vi "SWERVE DRIVE AUTO.vi"(8 "error in (no error)":errorcluster, 11 "auto pgm array":T4[](array[typedef])=[{"auto drive command"={"TRANSLATE"={"drive\ndistance (ft)"=10.0, "steer\nbearing (deg)"=0.0, "max strafe\nvelocity (ft/s)"=10.0, "max strafe\naccel (ft/s^2)"=58.7}, "ROTATE"={"rotate to\nbearing (deg)"=0.0, "max rotate\nvelocity (deg/s)"=0.0, "max rotate\naccel (ft/s^2)"=25.0}}, "sub-systems"={"start INTAKE"=FALSE, "extend FLAP"=FALSE, "SHOOT"=FALSE, "retract FLAP"=FALSE, "TARGET SPEAKER"=FALSE, "TARGET AMP"=FALSE, "TARGET OFF"=FALSE, "DANCE"=FALSE}}, {"auto drive command"={"TRANSLATE"={"drive\ndistance (ft)"=5.0, "steer\nbearing (deg)"=180.0, "max strafe\nvelocity (ft/s)"=5.0, "max strafe\naccel (ft/s^2)"=58.7}, "ROTATE"={"rotate to\nbearing (deg)"=0.0, "max rotate\nvelocity (deg/s)"=180.0, "max rotate\naccel (ft/s^2)"=25.0}}, "sub-systems"={"start INTAKE"=FALSE, "extend FLAP"=FALSE, "SHOOT"=FALSE, "retract FLAP"=FALSE, "TARGET SPEAKER"=FALSE, "TARGET AMP"=FALSE, "TARGET OFF"=FALSE, "DANCE"=FALSE}}] {"auto drive command"."ROTATE"."max rotate\naccel (ft/s^2)" min=0.0 max=200.0 step=0.1 format="%_3f"; "auto drive command"."ROTATE"."max rotate\nvelocity (deg/s)" min=0.0 step=0.001; "auto drive command"."TRANSLATE"."max strafe\naccel (ft/s^2)" min=0.0 max=200.0 step=0.1 format="%_3f"; "auto drive command"."TRANSLATE"."max strafe\nvelocity (ft/s)" min=0.0 max=20.0 step=0.001 format="%_5f"}) -> (0 "error out":errorcluster)   [LabVIEW 2023]
uses:
  ctrl defs/ctrl AUTONOMOUS step control.ctl
  ctrl defs/ctrl AUTONOMOUS drive step control.ctl
  ctrl defs/ctrl AUTONOMOUS systems step control.ctl
  ctrl defs/ctrl AUTO STATES.ctl
  <vilib>/Rock Robotics/WPI/ThirdParty/REV Robotics/REVLib/Typedef/Spark MAX Smart Motion Parameters.ctl
  <vilib>/Rock Robotics/WPI/ThirdParty/REV Robotics/REVLib/Typedef/Spark MAX Control Type.ctl
  Global INIT.vi
  Global odometry.vi
  <vilib>/Rock Robotics/WPI/ThirdParty/Phoenix-LabVIEW/CANCoder/Get/CTRE_Phoenix_CANcoder_GetSensorData.vi
  Global stack names.vi
  <vilib>/Rock Robotics/Network Tables/NT Read Boolean.vi
  <vilib>/Rock Robotics/Network Tables/NT Write Boolean.vi
panel:
  out "Sensor Velocity":dbl[](array[numeric])
  in  "Smart Motion Parameters":T1
  in  "PID Constants":T2={"P Gain"=0.0, "I Gain"=0.0, "D Gain"=0.0, "F Gain"=0.0, "I Zone"=0.0, "Min Output"=-1.0, "Max Output"=1.0} {"Max Output" min=0.0 max=1.0 step=0.01; "Min Output" min=-1.0 max=0.0 step=0.01}
  in  "loop exit":bool
  in  "STATE":T3
  out "wheel\npos (rev)":dbl[](array[numeric])
  out "@ target":bool[](array[boolean])
  out "pos\ntarget (rev)":dbl[](array[numeric])
  out "rev tol\nto target":dbl
  out "distance (ft)\nto wheel revs":dbl
  out "vel to wheel\nspeed\n(rpm per ft/s)":dbl
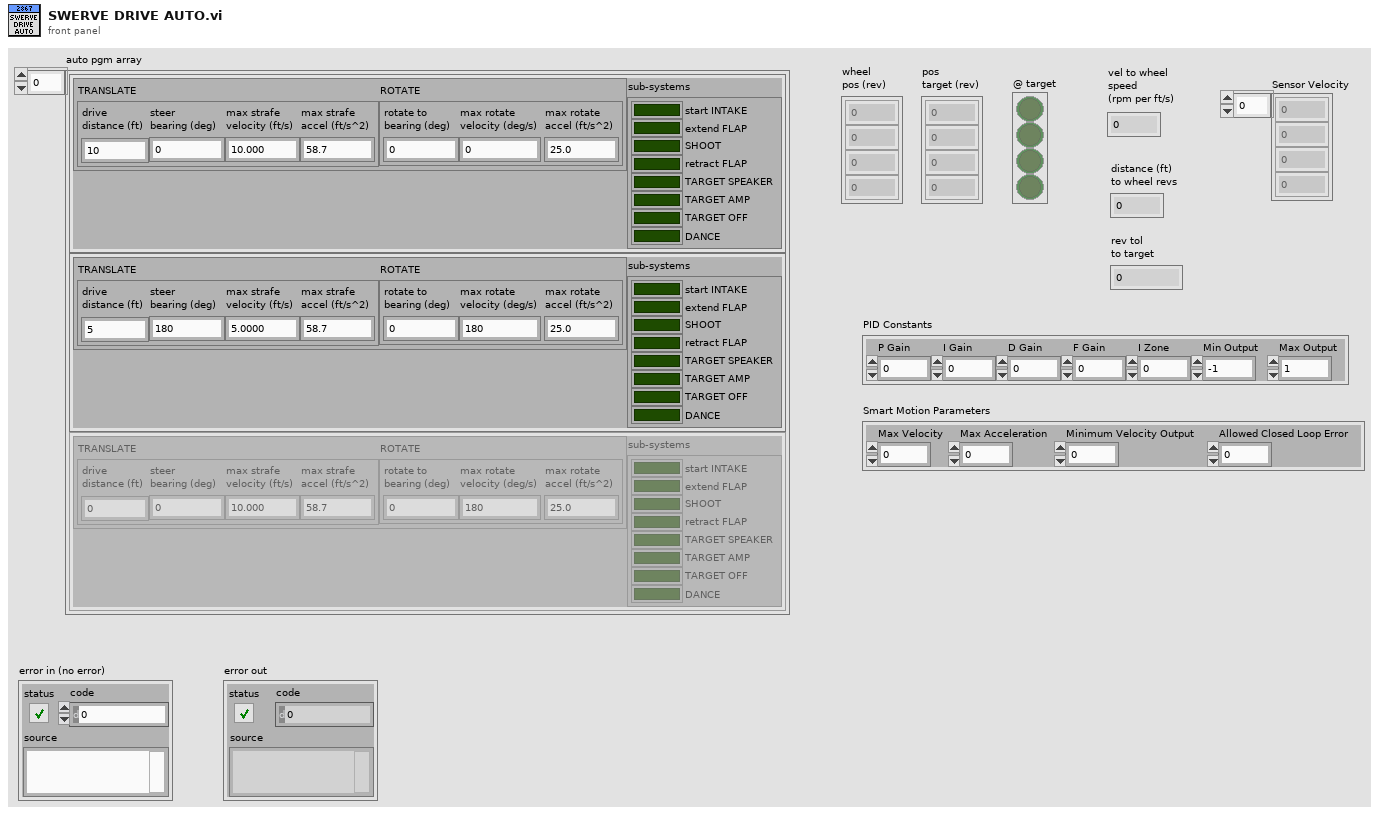
[diagram p1: front panel]
types:
  T1 = typedef "Spark MAX Smart Motion Parameters.ctl" = cluster{"Max Velocity":dbl, "Max Acceleration":dbl, "Minimum Velocity Output":dbl, "Allowed Closed Loop Error":dbl}
  T2 = cluster{"P Gain":dbl, "I Gain":dbl, "D Gain":dbl, "F Gain":dbl, "I Zone":dbl, "Min Output":dbl, "Max Output":dbl}
  T3 = typedef "ctrl AUTO STATES.ctl" = enum16{"TRANSLATE", "ROTATE", "TARGET", "INTAKE", "SHOOT", "DANCE", "WAIT for INTAKE", "WAIT for SHOOTER", "END", "SUB-SYSTEMS"}
  T4 = typedef "ctrl AUTONOMOUS step control.ctl" = cluster{"auto drive command":T5, "sub-systems":T6}
  T5 = typedef "ctrl AUTONOMOUS drive step control.ctl" = cluster{"TRANSLATE":cluster{"drive\ndistance (ft)":dbl, "steer\nbearing (deg)":dbl, "max strafe\nvelocity (ft/s)":dbl, "max strafe\naccel (ft/s^2)":dbl}, "ROTATE":cluster{"rotate to\nbearing (deg)":dbl, "max rotate\nvelocity (deg/s)":dbl, "max rotate\naccel (ft/s^2)":dbl}}
  T6 = typedef "ctrl AUTONOMOUS systems step control.ctl" = cluster{"start INTAKE":bool, "extend FLAP":bool, "SHOOT":bool, "retract FLAP":bool, "TARGET SPEAKER":bool, "TARGET AMP":bool, "TARGET OFF":bool, "DANCE":bool}
  T7 = typedef "ctrl swerve motor.ctl" = cluster{"description":string, "MOTOR SELECT":T8, "Installed?":bool, "CAN ID":u8, "refnum name":string, "Invert":bool, "Idle Mode":T9, "Current limiting":T10, "MOTOR PIDF coefficients":T11, "gear ratio":dbl}
  T8 = typedef "ctrl MOTOR SELECT.ctl" = i16
  T9 = typedef "Spark MAX Idle Mode.ctl" = enum16{"Coast", "Brake"}
  T10 = typedef "ctrl Spark MAX current limiting.ctl" = cluster{"Linearized":bool, "Free Speed (A)":dbl, "Primay (A)":dbl, "Limit RPM (0)":u32}
  T11 = typedef "ctrl motor PIDF coefficients.ctl" = cluster{"PIDF":cluster{"P Gain":dbl, "I Gain":dbl, "D Gain":dbl, "F Gain":dbl, "I Zone":dbl, "Min Output":dbl, "Max Output":dbl}, "Smart Motion":T1}
  T12 = typedef "ctrl swerve module.ctl" = cluster{"descr":string, "V":dbl, "POS":dbl, "target":dbl, "ABS":dbl, "from pivot to module":cluster{"R":dbl, "theta (deg)":dbl, "theta spin (deg)":dbl, "theta park (deg)":dbl}, "coord wrt geom CTR":cluster{"X":dbl, "Y":dbl}, "corner wt (lbm)":dbl}
  T13 = typedef "WPI_MotorControlDeviceRef.ctl" = cluster{"DeviceStatus":errorcluster, "Type":T14, "PWM":cluster{"PWM Channel":T15, "DeadBand":T16}, "CAN":cluster{"Device Number":u8, "SetOutput VI Ref":variant, "GetOutput VI Ref":variant, "Enable VI Ref":variant, "Disable VI Ref":variant, "Data":variant}, "Invert":bool, "DIO PWM":cluster{"PWM \"Enable\" Channel":T15, "DIOChannel":T17, "PWM Rate":dbl}}
  T14 = typedef "WPI_MotorControlType.ctl" = enum16{"PWM", "CAN", "DIO PWM"}
  T15 = typedef "FPGA_DIOPWMChannel.ctl" = enum8{"PWM 0", "PWM 1", "PWM 2", "PWM 3", "PWM 4", "PWM 5", "PWM 6", "PWM 7", "PWM 8", "PWM 9", "PWM MXP 0", "PWM MXP 1", "PWM MXP 2", "PWM MXP 3", "PWM MXP 4", "PWM MXP 5", "PWM MXP 6", "PWM MXP 7", "PWM MXP 8", "PWM MXP 9", "Invalid"}
  T16 = typedef "WPI_PWMDeadband.ctl" = cluster{"Name":string, "maxPositivePwm":i32, "minPositivePwm":i32, "centerPwm":i32, "maxNegativePwm":i32, "minNegativePwm":i32, "angularRange":u16}
  T17 = typedef "FPGA_DIOChannel.ctl" = enum8{"DIO 0", "DIO 1", "DIO 2", "DIO 3", "DIO 4", "DIO 5", "DIO 6", "DIO 7", "DIO 8", "DIO 9", "DIO MXP 0", "DIO MXP 1", "DIO MXP 2", "DIO MXP 3", "DIO MXP 4", "DIO MXP 5", "DIO MXP 6", "DIO MXP 7", "DIO MXP 8", "DIO MXP 9", "DIO MXP 10", "DIO MXP 11", "DIO MXP 12", "DIO MXP 13", "DIO MXP 14", "DIO MXP 15", "SPI Port CS1", "SPI Port CS2", "SPI Port CS3", "SPI Port MISO", "SPI Port MOSI", "Invalid"}
  T18 = typedef "CTRE_Phoenix_CANcoder_DeviceRef.ctl" = cluster{"DeviceStatus":errorcluster, "Device Number":u8, "Handle":u64, "UsageFrame":u32, "Library Path":path}
  T19 = cluster{"Driver":T13, "Steer":T13, "Encoder":T18}[]
  T20 = typedef "Spark MAX Control Type.ctl" = enum16{"Percent VBus", "Voltage", "Velocity", "Position", "Smart Motion", "Current", "Smart Velocity"}
  T21 = typedef "ctrl stack - INTAKE SHOOTER.ctl" = cluster{"INTAKE STATE":string, "RUN INTAKE?":string, "RUN REVERSE?":string, "NOTE LOADED?":string, "SHOOTER STATE":string, "SHOOTER FIRE?":string, "SHOOT AMP?":string, "EXTEND FLAP?":string, "LOOKING for NOTE":string, "OVERIDE NOTE CHECK":string}
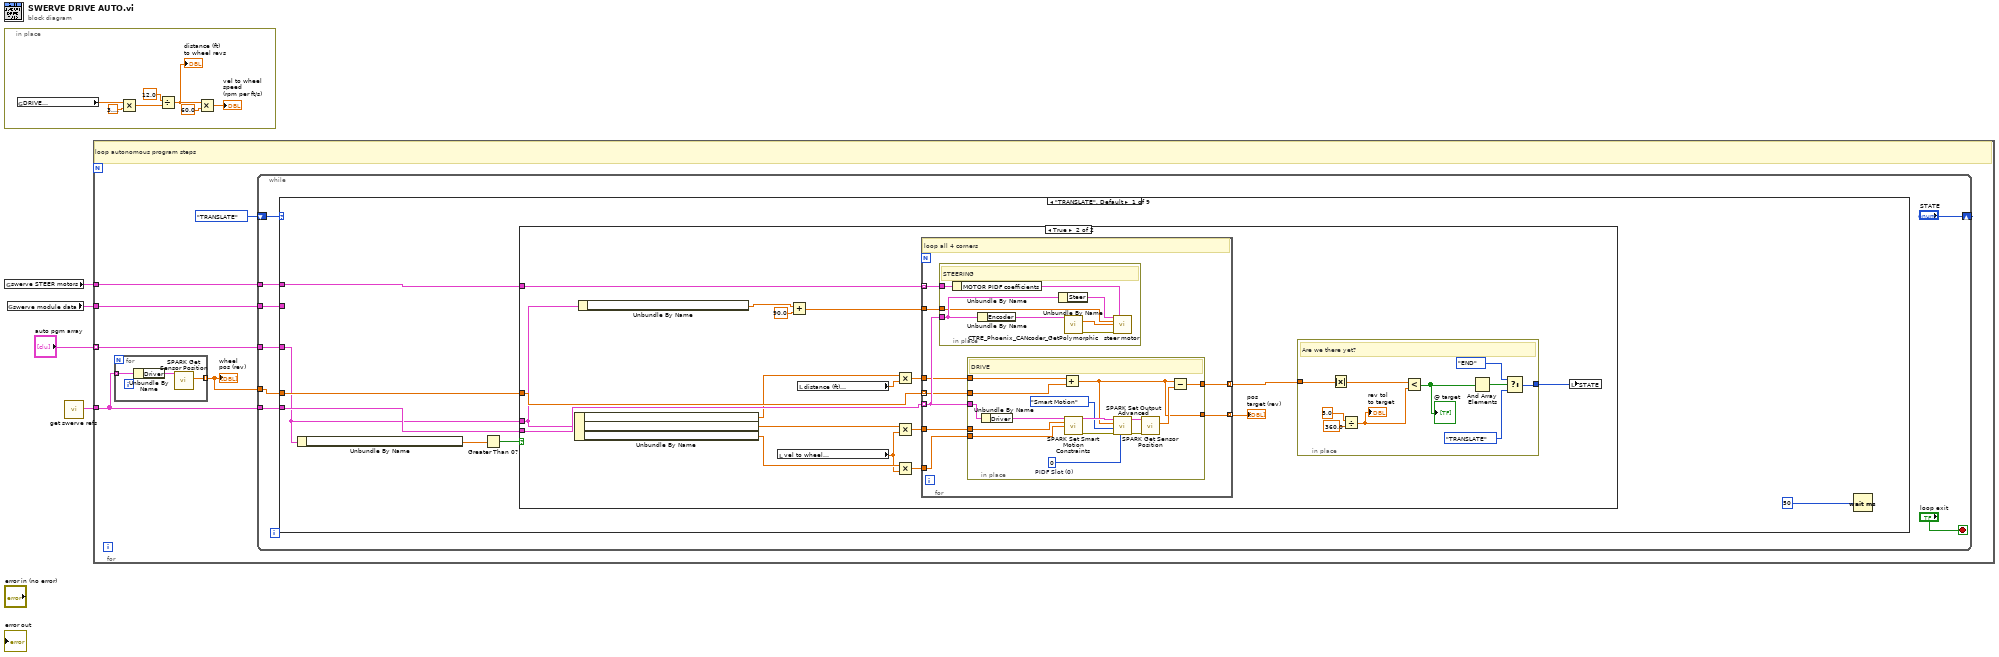
[diagram p0: block diagram]
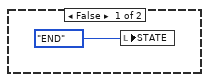
[diagram p2: hidden frame]
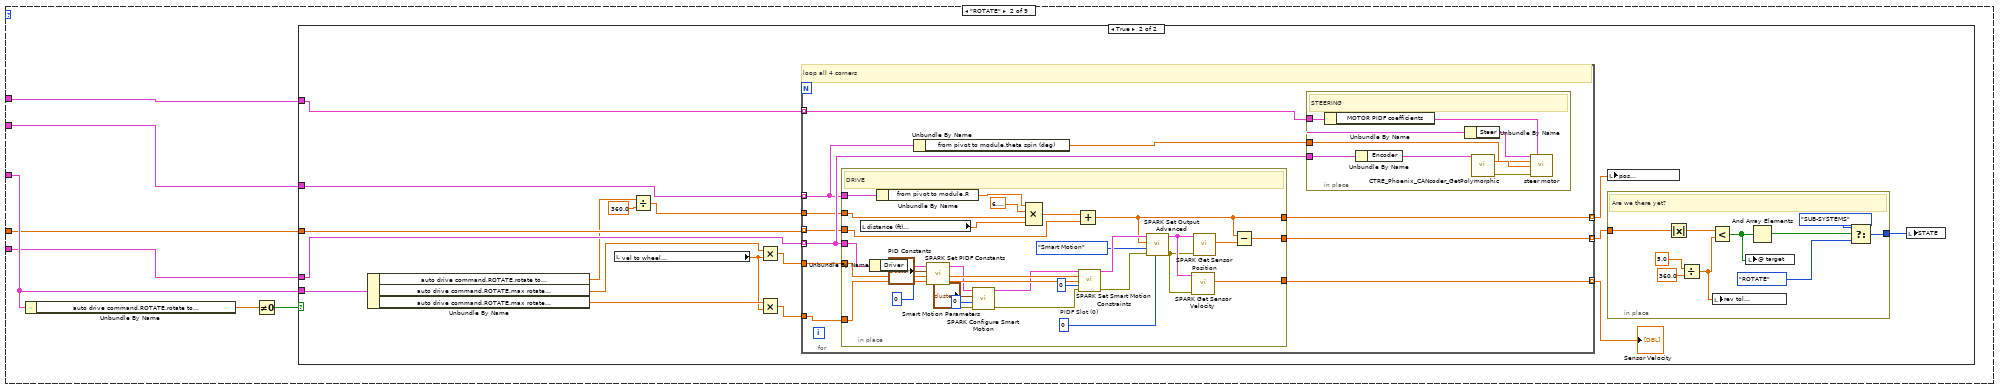
[diagram p3: hidden frame]
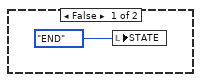
[diagram p4: hidden frame]
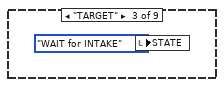
[diagram p5: hidden frame]
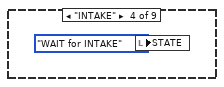
[diagram p6: hidden frame]
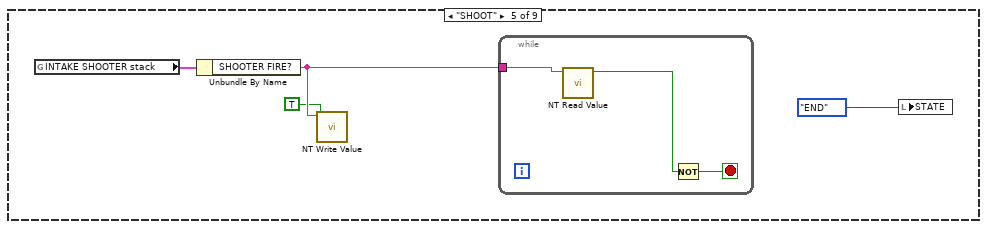
[diagram p7: hidden frame]
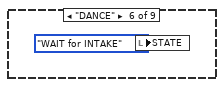
[diagram p8: hidden frame]
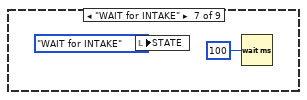
[diagram p9: hidden frame]
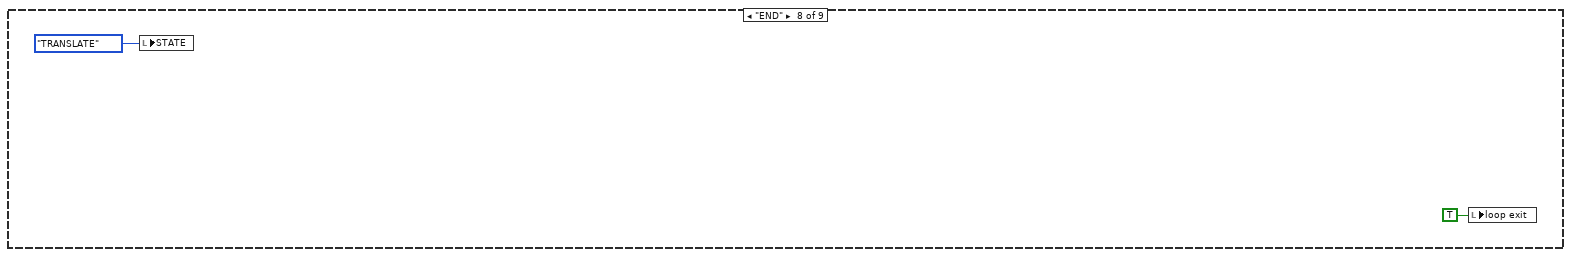
[diagram p10: hidden frame]
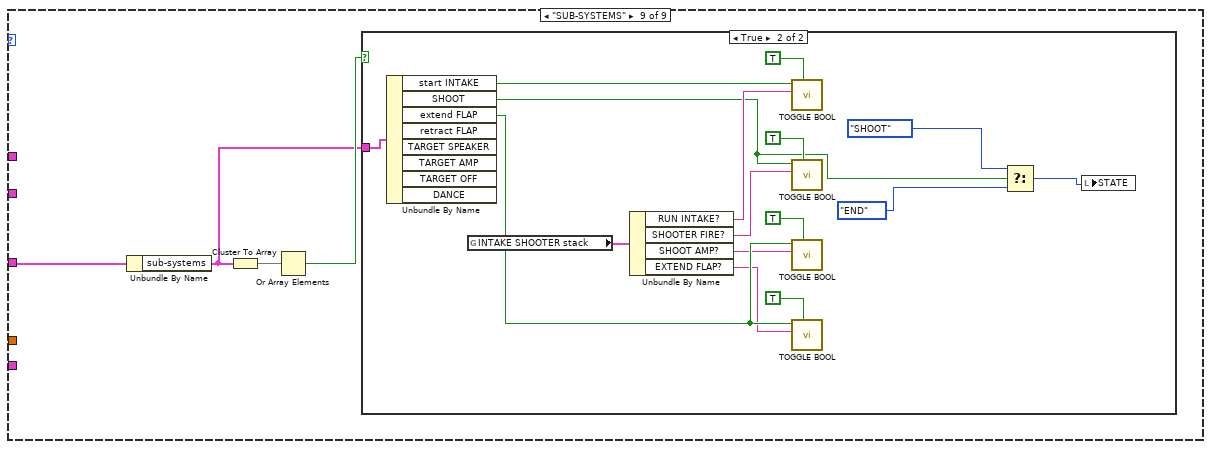
[diagram p11: hidden frame]
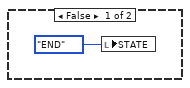
[diagram p12: hidden frame]
diagram:
  n1 = in-place {
    n2 = global read "Global INIT.vi" "DRIVE\nwheel diam (in)"() -> (w11:dbl)
    n3 = Multiply(x=w11, y=3.141592653589793) -> (x*y=w8:dbl)
    n4 = Divide(x=12.0, y=w8) -> (x/y=w7:dbl)
    "distance (ft)\nto wheel revs" <- w7
    n5 = Multiply(x=w7, y=60.0) -> (x*y=→"vel to wheel\nspeed\n(rpm per ft/s)":dbl)
  }
  n6 = global read "Global INIT.vi" "swerve STEER motors"() -> (w2:T7[])
  n7 = global read "Global odometry.vi" "swerve module data"() -> (w1:T12[])
  n8 = call "get swerve refs.vi"() -> ("Swerve refs"=w3:T19)  [unwired: 10 in, 1 out]
  n9 = for {
    tunnel: "auto pgm array" -> [w15] mode=indexing
    tunnel: w3 -> [w14]
    tunnel: w2 -> [w13]
    tunnel: w1 -> [w12]
    # "loop autonomous program steps"
    n10 = for {
      tunnel: w14 -> [w215] mode=indexing
      tunnel: [w213] -> w16 mode=indexing
      n11 = Unbundle By Name(w215) -> ("Driver"=w214:T13)
      n12 = call <vilib>:"SPARK Get Sensor Position.vi"("MotorControlDevRef in"=w214) -> ("Sensor Position"=w213:dbl)  [unwired: 7 in, 3 out]
    }
    "wheel\npos (rev)" <- w16
    n13 = while {
      shift-right: ["STATE"] -> _
      shift-left: ctrl_AUTO_STATES."TRANSLATE" -> [w25]
      tunnel: w16 -> [w22]
      tunnel: w15 -> [w24]
      tunnel: w14 -> [w23]
      tunnel: w13 -> [w21]
      tunnel: w12 -> [w20]
      stop <- "loop exit" stop-if-true
      n14 = case shown="\"TRANSLATE\", Default" w25 {
        tunnel: w24 -> [w27 w98 _ _ _ _ _ _ w195]
        tunnel: w23 -> [w30 w97 _ _ _ _ _ _ _]
        tunnel: w22 -> [w29 w96 _ _ _ _ _ _ _]
        tunnel: w21 -> [w28 w95 _ _ _ _ _ _ _]
        tunnel: w20 -> [_ w94 _ _ _ _ _ _ _]
        frame "TRANSLATE", Default {
          n15 = Unbundle By Name(w27) -> ("auto drive command.TRANSLATE.drive\ndistance (ft)"=w32:dbl)
          n16 = Greater Than 0?(x=w32) -> (x > 0?=w31:bool)
          n17 = case shown="True" w31 {
            tunnel: w30 -> [_ w51]
            tunnel: w29 -> [_ w50]
            tunnel: w28 -> [_ w49]
            tunnel: w27 -> [_ w48]
            frame False {
              n18 = local write "STATE"(ctrl_AUTO_STATES."END") -> ()
            }
            frame True {
              n19 = Unbundle By Name(w48) -> ("auto drive command.TRANSLATE.drive\ndistance (ft)"=w44:dbl, "auto drive command.TRANSLATE.max strafe\nvelocity (ft/s)"=w43:dbl, "auto drive command.TRANSLATE.max strafe\naccel (ft/s^2)"=w38:dbl)
              n20 = Unbundle By Name(w48) -> ("auto drive command.TRANSLATE.steer\nbearing (deg)"=w47:dbl)
              n21 = local read "vel to wheel\nspeed\n(rpm per ft/s)"() -> (w37:dbl)
              n22 = Add(x=w47, y=90.0) -> (x+y=w45:dbl)
              n23 = local read "distance (ft)\nto wheel revs"() -> (w42:dbl)
              n24 = Multiply(x=w44, y=w42) -> (x*y=w41:dbl)
              n25 = Multiply(x=w43, y=w37) -> (x*y=w40:dbl)
              n26 = Multiply(x=w38, y=w37) -> (x*y=w39:dbl)
              n27 = for {
                tunnel: w51 -> [w68] mode=indexing
                tunnel: w50 -> [w64] mode=indexing
                tunnel: w49 -> [w69] mode=indexing
                tunnel: w45 -> [w70]
                tunnel: w41 -> [w67]
                tunnel: w40 -> [w65]
                tunnel: w39 -> [w66]
                tunnel: [w63] -> w36 mode=indexing
                tunnel: [w62] -> w35 mode=indexing
                # "loop all 4 corners"
                n28 = in-place {
                  in-place-border: w68 -> [w90]
                  in-place-border: w70 -> [w89]
                  in-place-border: w69 -> [w87]
                  # "STEERING"
                  n29 = Unbundle By Name(w87) -> ("MOTOR PIDF coefficients"=w86:T11)
                  n30 = Unbundle By Name(w90) -> ("Encoder"=w93:T18)
                  n31 = Unbundle By Name(w90) -> ("Steer"=w91:T13)
                  n32 = call-poly <vilib>:"CTRE_Phoenix_CANcoder_GetPolymorphic.vi"("CTRE_CANcoder_DeviceRef"=w93) -> ("Position"=w92:dbl, "error out"=w88:errorcluster)  [unwired: 10 in, 3 out]
                  n33 = call "steer motor.vi"("MotorControlDevRef"=w91, "MOTOR PIDF coefficients"=w86, "target"=w89, "encoder"=w92, "error in (no error)"=w88) -> ()  [unwired: 10 in, 1 out]
                }
                n34 = in-place {
                  in-place-border: w68 -> [w81]
                  in-place-border: w67 -> [w79]
                  in-place-border: w66 -> [w77]
                  in-place-border: w65 -> [w78]
                  in-place-border: w64 -> [w76]
                  in-place-border: [w72] -> w63
                  in-place-border: [w71] -> w62
                  w82 = 0  # PIDF Slot (0)
                  # "DRIVE"
                  n35 = Unbundle By Name(w81) -> ("Driver"=w80:T13)
                  n36 = Add(x=w79, y=w76) -> (x+y=w71:dbl)
                  n37 = call <vilib>:"SPARK Set Smart Motion Constraints.vi"("MotorControlDeviceRef"=w80, "Max Velocity"=w78, "Max Acceleration"=w77) -> ("MotorControlDeviceRef"=w84:T13, "error out"=w85:errorcluster)  [unwired: 11 in]
                  n38 = call <vilib>:"SPARK Set Output Advanced.vi"("PIDF Slot (0)"=w82, "error in (no error)"=w85, "Control Mode"=Spark_MAX_Control_Type."Smart Motion", "Setpoint"=w71, "MotorControlDevRef"=w84) -> ("error out"=w75:errorcluster, "MotorControlDevRef"=w74:T13)  [unwired: 5 in]
                  n39 = call <vilib>:"SPARK Get Sensor Position.vi"("error in (no error)"=w75, "MotorControlDevRef in"=w74) -> ("Sensor Position"=w73:dbl)  [unwired: 6 in, 3 out]
                  n40 = Subtract(x=w71, y=w73) -> (x-y=w72:dbl)
                }
              }
              "pos\ntarget (rev)" <- w35
              n41 = in-place {
                in-place-border: w36 -> [w61]
                in-place-border: [w57] -> w34
                # "Are we there yet?"
                n42 = Absolute Value(x=w61) -> (abs(x)=w56:dbl[])
                n43 = Divide(x=5.0, y=360.0) -> (x/y=w55:dbl)
                "rev tol\nto target" <- w55
                n44 = Less?(x=w56, y=w55) -> (x < y?=w52:bool[])
                "@ target" <- w52
                n45 = And Array Elements(Boolean array=w52) -> (logical AND=w60:bool)
                n46 = Select(t=ctrl_AUTO_STATES."END", s=w60, f=ctrl_AUTO_STATES."TRANSLATE") -> (s? t:f=w57:T3)
              }
              n47 = local write "STATE"(w34) -> ()
            }
          }
          n48 = Wait (ms)(milliseconds to wait=u32 50) -> ()  [unwired: 1 out]
        }
        frame "ROTATE" {
          n49 = Unbundle By Name(w98) -> ("auto drive command.ROTATE.rotate to\nbearing (deg)"=w100:dbl)
          n50 = Not Equal To 0?(x=w100) -> (x != 0?=w99:bool)
          n51 = case shown="True" w99 {
            tunnel: w97 -> [_ w118]
            tunnel: w96 -> [_ w117]
            tunnel: w95 -> [_ w116]
            tunnel: w98 -> [_ w115]
            tunnel: w94 -> [_ w108]
            frame False {
              n52 = local write "STATE"(ctrl_AUTO_STATES."END") -> ()
            }
            frame True {
              n53 = Unbundle By Name(w115) -> ("auto drive command.ROTATE.rotate to\nbearing (deg)"=w107:dbl, "auto drive command.ROTATE.max rotate\nvelocity (deg/s)"=w114:dbl, "auto drive command.ROTATE.max rotate\naccel (ft/s^2)"=w111:dbl)
              n54 = local read "vel to wheel\nspeed\n(rpm per ft/s)"() -> (w110:dbl)
              n55 = Divide(x=w107, y=360.0) -> (x/y=w105:dbl)
              n56 = Multiply(x=w114, y=w110) -> (x*y=w113:dbl)
              n57 = Multiply(x=w111, y=w110) -> (x*y=w112:dbl)
              n58 = for {
                tunnel: w118 -> [w138] mode=indexing
                tunnel: w117 -> [w135] mode=indexing
                tunnel: w116 -> [w139] mode=indexing
                tunnel: w113 -> [w136]
                tunnel: w112 -> [w137]
                tunnel: [w134] -> w109 mode=indexing
                tunnel: [w133] -> w104 mode=indexing
                tunnel: w108 -> [w131] mode=indexing
                tunnel: w105 -> [w130]
                tunnel: [w129] -> w102 mode=indexing
                # "loop all 4 corners"
                n59 = in-place {
                  in-place-border: w138 -> [w165]
                  in-place-border: w137 -> [w162]
                  in-place-border: w136 -> [w163]
                  in-place-border: w135 -> [w161]
                  in-place-border: [w159] -> w134
                  in-place-border: [w158] -> w133
                  in-place-border: w131 -> [w157]
                  in-place-border: w130 -> [w154]
                  in-place-border: [w140] -> w129
                  w166 = 0  # PIDF Slot (0)
                  # "DRIVE"
                  n60 = local read "distance (ft)\nto wheel revs"() -> (w153:dbl)
                  n61 = Unbundle By Name(w165) -> ("Driver"=w164:T13)
                  n62 = Unbundle By Name(w157) -> ("from pivot to module.R"=w156:dbl)
                  n63 = call <vilib>:"SPARK Set PIDF Constants.vi"("PIDF Slot"=0, "PID Constants"="PID Constants", "MotorControlDeviceRef"=w164) -> ("error out"=w147:errorcluster, "MotorControlDeviceRef"=w149:T13)  [unwired: 7 in]
                  n64 = call <vilib>:"SPARK Configure Smart Motion.vi"("error in"=w147, "PIDF Slot (0)"=0, "Smart Motion Parameters"="Smart Motion Parameters", "MotorControlDeviceRef"=w149) -> ("error out"=w146:errorcluster, "MotorControlDeviceRef"=w148:T13)  [unwired: 6 in]
                  n65 = Compound Arithmetic op=MULTIPLY(w156, 6.283185307179586, w154, w153) -> (w152:dbl)
                  n66 = Add(x=w152, y=w161) -> (x+y=w158:dbl)
                  n67 = call <vilib>:"SPARK Set Smart Motion Constraints.vi"("MotorControlDeviceRef"=w148, "Max Velocity"=w163, "Max Acceleration"=w162, "PIDF Slot (0)"=0, "error in"=w146) -> ("MotorControlDeviceRef"=w168:T13, "error out"=w169:errorcluster)  [unwired: 9 in]
                  n68 = call <vilib>:"SPARK Set Output Advanced.vi"("PIDF Slot (0)"=w166, "error in (no error)"=w169, "Control Mode"=Spark_MAX_Control_Type."Smart Motion", "Setpoint"=w158, "MotorControlDevRef"=w168) -> ("error out"=w141:errorcluster, "MotorControlDevRef"=w142:T13)  [unwired: 5 in]
                  n69 = call <vilib>:"SPARK Get Sensor Velocity.vi"("error in (no error)"=w141, "MotorControlDevRef in"=w142) -> ("Sensor Velocity"=w140:dbl)  [unwired: 6 in, 3 out]
                  n70 = call <vilib>:"SPARK Get Sensor Position.vi"("error in (no error)"=w141, "MotorControlDevRef in"=w142) -> ("Sensor Position"=w160:dbl)  [unwired: 6 in, 3 out]
                  n71 = Subtract(x=w158, y=w160) -> (x-y=w159:dbl)
                }
                n72 = Unbundle By Name(w131) -> ("from pivot to module.theta spin (deg)"=w132:dbl)
                n73 = in-place {
                  in-place-border: w138 -> [w174]
                  in-place-border: w139 -> [w172]
                  in-place-border: w132 -> [w170]
                  # "STEERING"
                  n74 = Unbundle By Name(w172) -> ("MOTOR PIDF coefficients"=w171:T11)
                  n75 = Unbundle By Name(w174) -> ("Encoder"=w177:T18)
                  n76 = Unbundle By Name(w174) -> ("Steer"=w175:T13)
                  n77 = call-poly <vilib>:"CTRE_Phoenix_CANcoder_GetPolymorphic.vi"("CTRE_CANcoder_DeviceRef"=w177) -> ("Position"=w176:dbl, "error out"=w173:errorcluster)  [unwired: 10 in, 3 out]
                  n78 = call "steer motor.vi"("MotorControlDevRef"=w175, "MOTOR PIDF coefficients"=w171, "target"=w170, "encoder"=w176, "error in (no error)"=w173) -> ()  [unwired: 10 in, 1 out]
                }
              }
              "Sensor Velocity" <- w102
              n79 = local write "pos\ntarget (rev)"(w104) -> ()
              n80 = in-place {
                in-place-border: w109 -> [w128]
                in-place-border: [w124] -> w103
                # "Are we there yet?"
                n81 = Absolute Value(x=w128) -> (abs(x)=w123:dbl[])
                n82 = Divide(x=5.0, y=360.0) -> (x/y=w120:dbl)
                n83 = Less?(x=w123, y=w120) -> (x < y?=w119:bool[])
                n84 = local write "rev tol\nto target"(w120) -> ()
                n85 = local write "@ target"(w119) -> ()
                n86 = And Array Elements(Boolean array=w119) -> (logical AND=w127:bool)
                n87 = Select(t=ctrl_AUTO_STATES."SUB-SYSTEMS", s=w127, f=ctrl_AUTO_STATES."ROTATE") -> (s? t:f=w124:T3)
              }
              n88 = local write "STATE"(w103) -> ()
            }
          }
        }
        frame "TARGET" {
          n89 = local write "STATE"(ctrl_AUTO_STATES."WAIT for INTAKE") -> ()
        }
        frame "INTAKE" {
          n90 = local write "STATE"(ctrl_AUTO_STATES."WAIT for INTAKE") -> ()
        }
        frame "SHOOT" {
          n91 = global read "Global stack names.vi" "INTAKE SHOOTER stack"() -> (w182:T21)
          n92 = Unbundle By Name(w182) -> ("SHOOTER FIRE?"=w181:string)
          n93 = call-poly <vilib>:"NT Write Value.vi"("value"=TRUE, "name"=w181) -> ()  [unwired: 9 in, 1 out]
          n94 = while {
            tunnel: w181 -> [w186]
            stop <- w184 stop-if-true
            n95 = call-poly <vilib>:"NT Read Value.vi"("name"=w186) -> ("value"=w185:bool)  [unwired: 8 in, 2 out]
            n96 = Not(x=w185) -> (.not. x?=w184:bool)
          }
          n97 = local write "STATE"(ctrl_AUTO_STATES."END") -> ()
        }
        frame "DANCE" {
          n98 = local write "STATE"(ctrl_AUTO_STATES."WAIT for INTAKE") -> ()
        }
        frame "WAIT for INTAKE" {
          n99 = local write "STATE"(ctrl_AUTO_STATES."WAIT for INTAKE") -> ()
          n100 = Wait (ms)(milliseconds to wait=u32 100) -> ()  [unwired: 1 out]
        }
        frame "END" {
          n101 = local write "STATE"(ctrl_AUTO_STATES."TRANSLATE") -> ()
          n102 = local write "loop exit"(TRUE) -> ()
        }
        frame "SUB-SYSTEMS" {
          n103 = Unbundle By Name(w195) -> ("sub-systems"=w192:T6)
          n104 = Cluster To Array(cluster=w192) -> (array=w194:bool[])
          n105 = Or Array Elements(Boolean array=w194) -> (logical OR=w193:bool)
          n106 = case shown="True" w193 {
            tunnel: w192 -> [_ w212]
            frame False {
              n107 = local write "STATE"(ctrl_AUTO_STATES."END") -> ()
            }
            frame True {
              n108 = Unbundle By Name(w212) -> ("start INTAKE"=w210:bool, "SHOOT"=w200:bool, "extend FLAP"=w211:bool)  [unwired: 5 out]
              n109 = global read "Global stack names.vi" "INTAKE SHOOTER stack"() -> (w209:T21)
              n110 = Unbundle By Name(w209) -> ("RUN INTAKE?"=w206:string, "SHOOTER FIRE?"=w207:string, "SHOOT AMP?"=w208:string, "EXTEND FLAP?"=w205:string)
              n111 = call "TOGGLE BOOL.vi"("force"=TRUE, "stack ref name"=w206, "Button Pressed?"=w210) -> ()  [unwired: 8 in, 1 out]
              n112 = call "TOGGLE BOOL.vi"("force"=TRUE, "stack ref name"=w207, "Button Pressed?"=w200) -> ()  [unwired: 8 in, 1 out]
              n113 = call "TOGGLE BOOL.vi"("force"=TRUE, "stack ref name"=w208, "Button Pressed?"=w211) -> ()  [unwired: 8 in, 1 out]
              n114 = call "TOGGLE BOOL.vi"("force"=TRUE, "stack ref name"=w205, "Button Pressed?"=w211) -> ()  [unwired: 8 in, 1 out]
              n115 = Select(t=ctrl_AUTO_STATES."SHOOT", s=w200, f=ctrl_AUTO_STATES."END") -> (s? t:f=w197:T3)
              n116 = local write "STATE"(w197) -> ()
            }
          }
        }
      }
    }
  }
